vi "Pre-Install Custom Action.vi"(10 "Variant":variant) -> (0 "error out":errorcluster)   [LabVIEW 2019]
uses:
  <vilib>/nisyscfg/Get Installed Components.vi
  <vilib>/nisyscfg/nisyscfg.lvlib
panel:
  # "Check for Vision Development Module"
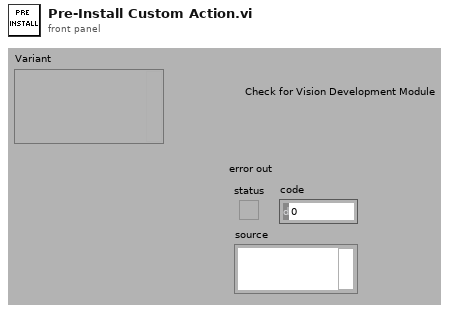
[diagram p1: front panel]
types:
  T1 = typedef "nisyscfg.lvlib/Software 1.2.ctl" = cluster{"title":string, "description":string, "ID":string, "version":string, "component type":T2}
  T2 = typedef "nisyscfg.lvlib/Component Type.ctl" = u32
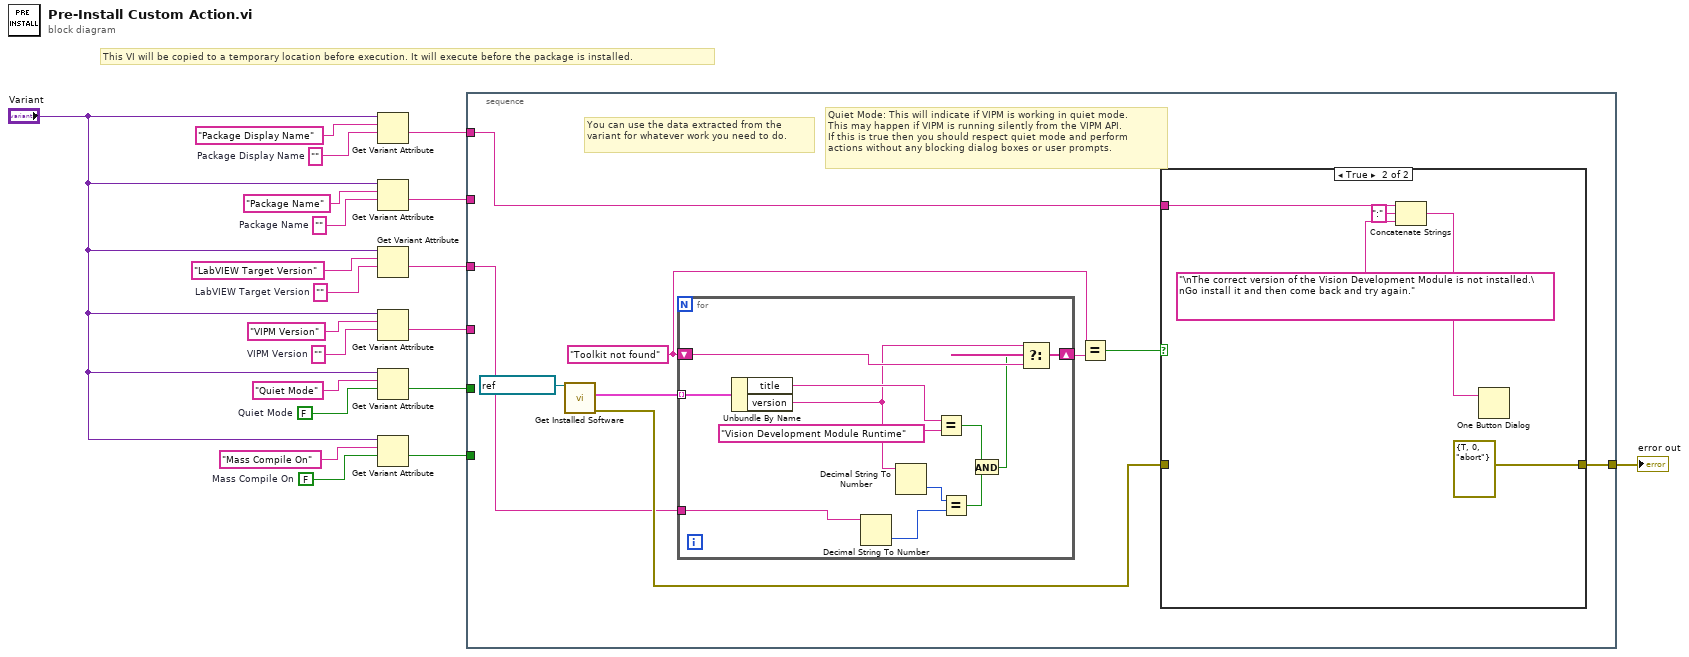
[diagram p0: block diagram]
diagram:
  w2 = FALSE  # Mass Compile On
  w4 = ""  # Package Display Name
  w11 = FALSE  # Quiet Mode
  w14 = ""  # VIPM Version
  w16 = ""  # LabVIEW Target Version
  w18 = ""  # Package Name
  # "This VI will be copied to a temporary location before execution. It will execute before the package is installed."
  n1 = Get Variant Attribute(Variant="Variant", name="Package Display Name", default value (empty Variant)=w4) -> (value=w10:string)  [unwired: 1 in, 3 out]
  n2 = Get Variant Attribute(Variant="Variant", name="Package Name", default value (empty Variant)=w18) -> (value=w9:string)  [unwired: 1 in, 3 out]
  n3 = Get Variant Attribute(Variant="Variant", name="LabVIEW Target Version", default value (empty Variant)=w16) -> (value=w8:string)  [unwired: 1 in, 3 out]
  n4 = Get Variant Attribute(Variant="Variant", name="VIPM Version", default value (empty Variant)=w14) -> (value=w7:string)  [unwired: 1 in, 3 out]
  n5 = Get Variant Attribute(Variant="Variant", name="Quiet Mode", default value (empty Variant)=w11) -> (value=w6:bool)  [unwired: 1 in, 3 out]
  n6 = Get Variant Attribute(Variant="Variant", name="Mass Compile On", default value (empty Variant)=w2) -> (value=w5:bool)  [unwired: 1 in, 3 out]
  n7 = stacked-sequence {
    tunnel: w10 -> [w22]
    tunnel: w9 -> [_]
    tunnel: w8 -> [w21]
    tunnel: w7 -> [_]
    tunnel: w6 -> [_]
    tunnel: w5 -> [_]
    tunnel: [w23] -> w1
    frame #0 {
      w25 = "Toolkit not found" ("version")
      # "Quiet Mode: This will indicate if VIPM is working in quiet mode.\nThis may happen if VIPM is running silently from the VIPM API.\nIf this is true then you should respect quiet mode and perform\nactions without any blocking dialog boxes or user prompts."
      # "You can use the data extracted from the variant for whatever work you need to do."
      n8 = call-poly <vilib>:"Get Installed Software.vi"("Session in"=refnum<k21> "localhost") -> ("error out"=w24:errorcluster, "Software Components"=w28:T1[])  [unwired: 8 in, 1 out]
      n9 = for {
        tunnel: w28 -> [w47] mode=indexing
        shift-right: [w44] -> w29
        shift-left: w25 -> [w43]
        tunnel: w21 -> [w39]
        n10 = Unbundle By Name(w47) -> ("title"=w45:string, "version"=w38:string)
        n11 = Decimal String To Number(string=w39) -> (number=w36:i32)  [unwired: 2 in, 1 out]
        n12 = Decimal String To Number(string=w38) -> (number=w37:i32)  [unwired: 2 in, 1 out]
        n13 = Equal?(x=w45, y="Vision Development Module Runtime" ("regular expression")) -> (x = y?=w42:bool)
        n14 = Equal?(x=w37, y=w36) -> (x = y?=w41:bool)
        n15 = And(x=w42, y=w41) -> (x .and. y?=w40:bool)
        n16 = Select(t=w38, s=w40, f=w43) -> (s? t:f=w44:string)
      }
      n17 = Equal?(x=w25, y=w29) -> (x = y?=w26:bool)
      n18 = case shown="True" w26 {
        tunnel: [w30 errorcluster {"status"=TRUE, "code"=0, "source"="abort"} ("error out")] -> w23
        tunnel: w24 -> [w30 _]
        tunnel: w22 -> [_ w33]
        frame False {
        }
        frame True {
          n19 = Concatenate Strings(w33, ":" ("string"), "\nThe correct version of the Vision Development Module is not installed.\nGo install it and then come back and try again." ("message")) -> (w31:string)
          n20 = One Button Dialog(message=w31) -> ()  [unwired: 1 in, 1 out]
        }
      }
    }
  }
  "error out" <- w1
